vi "Write Test.vi"(8 "error in (no error)":errorcluster, 10 "Test":refnum<class "Test.lvclass">[](array[class]), 11 "Bus in":refnum<class "Bus.lvclass">) -> (0 "error out":errorcluster, 3 "Bus out":refnum<class "Bus.lvclass">)   [LabVIEW 2014, in "Bus.lvclass"]
uses:
  Bus.lvclass
  TestClass/Test.lvclass
  Bus.lvclass/Bus.ctl
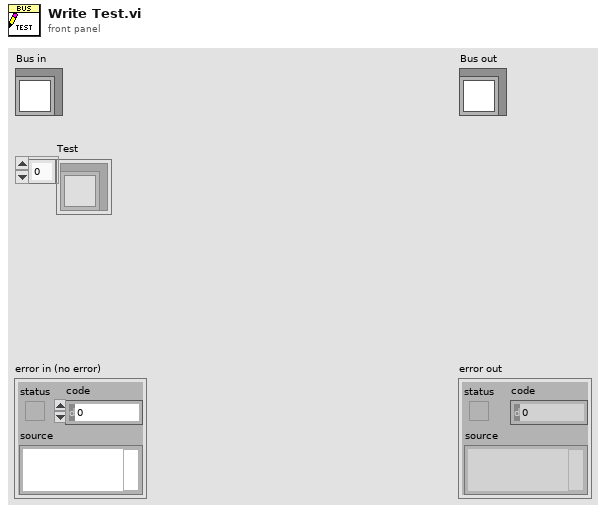
[diagram p1: front panel]
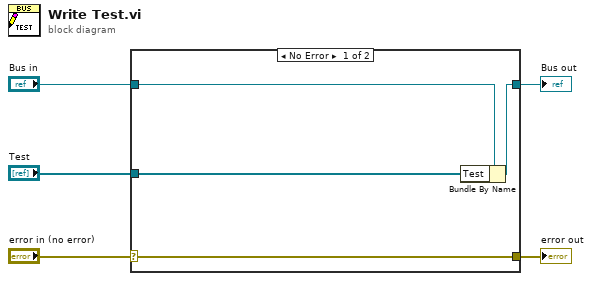
[diagram p0: block diagram]
diagram:
  n1 = case shown="No Error" "error in (no error)" {
    selector: "error in (no error)" -> [w9 w10]
    tunnel: [w9 w10] -> w4
    tunnel: [w7 w11] -> w2
    tunnel: "Bus in" -> [w8 w11]
    tunnel: "Test" -> [w6 _]
    frame No Error {
      n2 = Bundle By Name(cluster=w8, "Test"=w6) -> (w7:refnum<class "Bus.lvclass">)
    }
    frame Error {
    }
  }
  "error out" <- w4
  "Bus out" <- w2
